vi "Mover_motores_a_medida.vi"(6 "Ángulos de elementos ópticos:\nL2_in          L4_in        L4_out     P__out 2":dbl[](array[numeric]), 8 "Run":bool, 9 "Pasos por vuelta\nM1                 M2              M3            M4":dbl[](array[numeric])) -> ()   [LabVIEW 2013]
panel:
  in  "Argumento":string
  in  "Número de motor":string
  in  "Directorio scripts ArduinoStepper.py":path=path "C:/Users/franjas/Documents/rutinas-calibracion-slm"
  out "Pasos cada motor":dbl[](array[numeric])
  out "Valor mas cercano":dbl
  out "Angulo \nrecorrido":dbl
  out "Angulo por\npaso":dbl
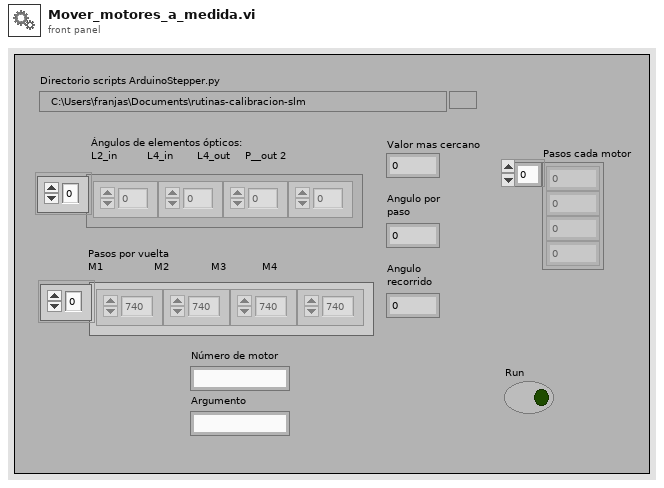
[diagram p1: front panel]
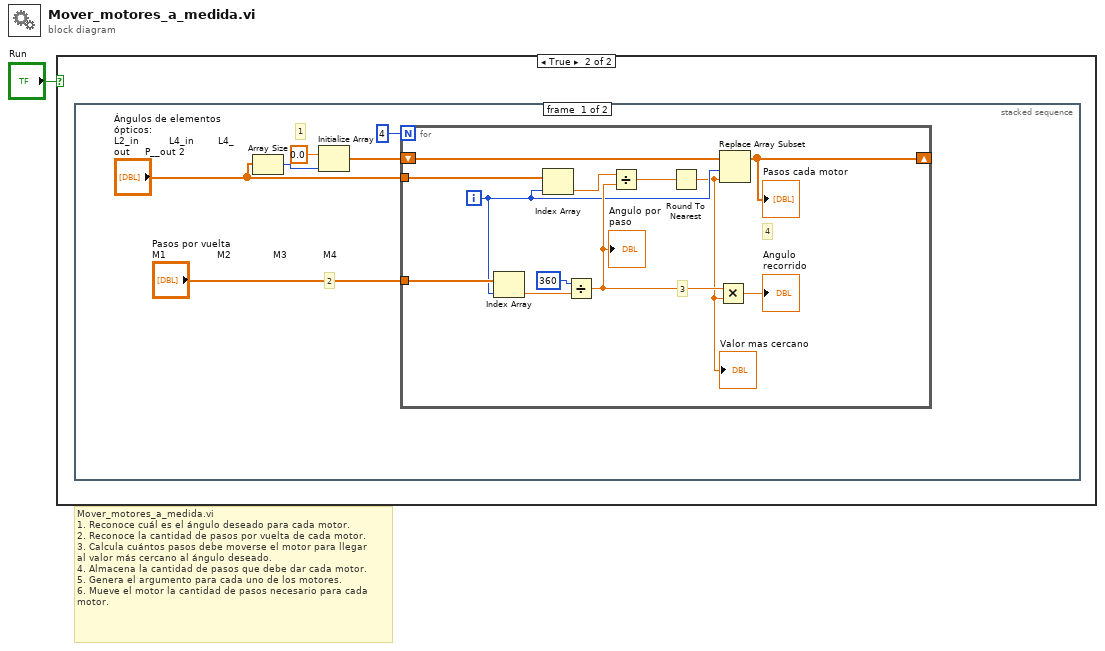
[diagram p0: block diagram]
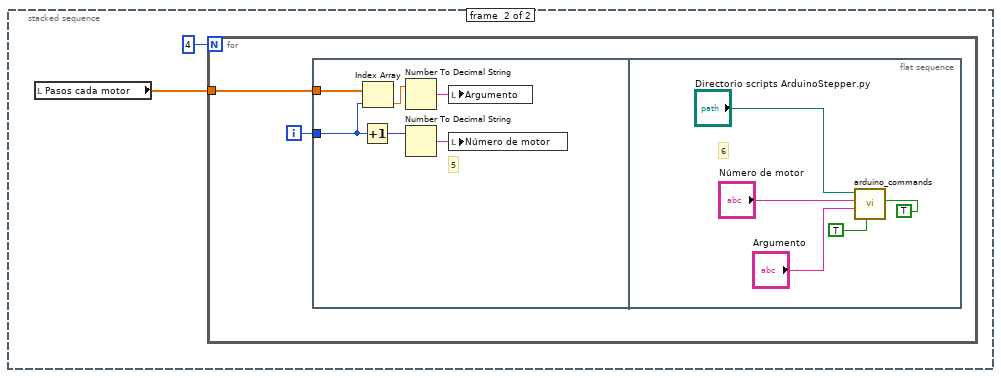
[diagram p3: hidden frame]
diagram:
  # "Mover_motores_a_medida.vi\n1. Reconoce cuál es el ángulo deseado para cada motor.\n2. Reconoce la cantidad de pasos por vuelta de cada motor.\n3. Calcula cuántos pasos debe moverse el motor para llegar\nal valor más cercano al ángulo deseado.\n4. Almacena la cantidad de pasos que debe dar cada motor.\n5. Genera el argumento para cada uno de los motores.\n6. Mueve el motor la cantidad de pasos necesario para cada\nmotor."
  n1 = case shown="True" "Run" {
    frame False {
    }
    frame True {
      n2 = stacked-sequence {
        frame #0 {
          # "2"
          # "1"
          n3 = Array Size(array="Ángulos de elementos ópticos:\nL2_in          L4_in        L4_out     P__out 2") -> (size(s)=w4:i32)
          n4 = Initialize Array(0.0 ("element"), w4) -> (w2:dbl[])
          n5 = for {
            N: 4 -> [_]
            tunnel: "Pasos por vuelta\nM1                 M2              M3            M4" -> [w15]
            tunnel: "Ángulos de elementos ópticos:\nL2_in          L4_in        L4_out     P__out 2" -> [w12]
            shift-right: [w8] -> _
            shift-left: w2 -> [w11]
            i -> [w10]
            # "4"
            # "3"
            n6 = Index Array(array=w15, index=w10) -> (element=w14:dbl)
            n7 = Index Array(array=w12, index=w10) -> (element=w13:dbl)
            n8 = Divide(x=360, y=w14) -> (x/y=w17:dbl)
            "Angulo por\npaso" <- w17
            n9 = Divide(x=w13, y=w17) -> (x/y=w18:dbl)
            n10 = Round To Nearest(number=w18) -> (nearest integer value=w9:dbl)
            "Valor mas cercano" <- w9
            n11 = Multiply(x=w17, y=w9) -> (x*y=→"Angulo \nrecorrido":dbl)
            n12 = Replace Array Subset(array=w11, new element=w9, index=w10) -> (w8:dbl[])
            "Pasos cada motor" <- w8
          }
        }
        frame #1 {
          n13 = local read "Pasos cada motor"() -> (w20:dbl[])
          n14 = for {
            N: 4 -> [_]
            tunnel: w20 -> [w23]
            i -> [w22]
            n15 = flat-sequence {
              tunnel: w23 -> [w29]
              tunnel: w22 -> [w24]
              frame #0 {
                # "5"
                n16 = Increment(x=w24) -> (x+1=w25:i32)
                n17 = Index Array(array=w29, index=w24) -> (element=w27:dbl)
                n18 = Number To Decimal String(number=w27) -> (decimal integer string=w28:string)  [unwired: 1 in]
                n19 = Number To Decimal String(number=w25) -> (decimal integer string=w26:string)  [unwired: 1 in]
                n20 = local write "Argumento"(w28) -> ()
                n21 = local write "Número de motor"(w26) -> ()
              }
              frame #1 {
                # "6"
                n22 = call "arduino_commands.vi"("Go to step"=TRUE, "Wait until completion? (T)"=TRUE ("wait until completion? (T)"), "Argumento"="Argumento", "Número de motor"="Número de motor", "Directorio scripts ArduinoStepper.py"="Directorio scripts ArduinoStepper.py") -> ()  [unwired: 6 in, 1 out]
              }
            }
          }
        }
      }
    }
  }
